vi "lvstyx_read.vi"(8 "error in (no error)":errorcluster, 10 "requested length":u16, 11 "file ptr":u32) -> (0 "error out":errorcluster, 1 "data":i8[](array[numeric]), 2 "actual length":u16, 3 "result":i32)   [LabVIEW 2010, in "lib1299.lvlib"]
uses:
  lib1299.lvlib
  cstyx/win32/cstyx.dll
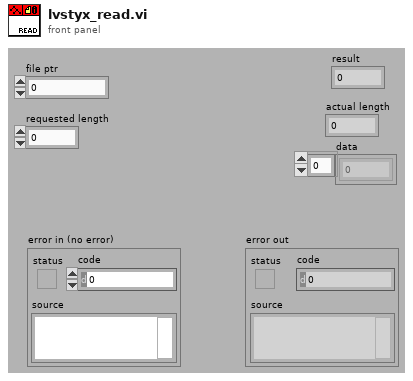
[diagram p1: front panel]
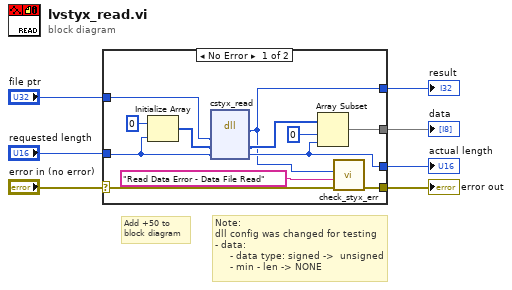
[diagram p0: block diagram]
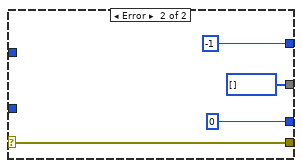
[diagram p2: hidden frame]
diagram:
  # "Add +50 to\nblock diagram"
  # "Note:\ndll config was changed for testing\n- data:\n     - data type: signed ->  unsigned\n     - min - len -> NONE"
  n1 = case shown="No Error" "error in (no error)" {
    selector: "error in (no error)" -> [w12 w23]
    tunnel: "file ptr" -> [w18 _]
    tunnel: [w11 w23] -> w5
    tunnel: "requested length" -> [w16 _]
    tunnel: [w9 u16 0 ("len")] -> w3
    tunnel: [w13 i8[] []] -> w2
    tunnel: [w8 -1 ("result")] -> w1
    frame No Error {
      n2 = Initialize Array(0, w16) -> (w17:i32[])
      n3 = dll-call lib="C:/work/ads1299evm/lib_1299/Styx/cstyx/win32/cstyx.dll" fn="cstyx_read"("file ptr"=w18, "data"=w17, "len"=w16) -> ("result"=w8:i32, "data"=w15:i8[], "len"=w9:u16)  [unwired: 4 in, 2 out]
      n4 = Array Subset(array=w15, index=0, length=w9) -> (w13:i8[])
      n5 = call "check_styx_err.vi"("error in (no error)"=w12, "Additional Comment"="Read Data Error - Data File Read", "return val"=w8) -> ("error out"=w11:errorcluster)  [unwired: 8 in]
    }
    frame Error {
    }
  }
  "error out" <- w5
  "result" <- w1
  "data" <- w2
  "actual length" <- w3
